vi "Lab Panel V5.28.vi"() -> ()   [LabVIEW 2013] (continued)
                            n2525 = Build Array("AMPS ON", "AMPS OFF", "VOLTS", "PF", "TEMP Live", "TEMP Neut", "CYCLE") -> (w4589:string[])
                            n2526 = Bundle By Name("Y"=w4612, "t0"=w4605) -> (w4604:waveform(dbl))  [unwired: 1 in]
                            n2527 = Bundle By Name("Y"=w4611, "t0"=w4605) -> (w4603:waveform(dbl))  [unwired: 1 in]
                            n2528 = Bundle By Name("Y"=w4610, "t0"=w4605) -> (w4602:waveform(dbl))  [unwired: 1 in]
                            n2529 = Bundle By Name("Y"=w4609, "t0"=w4605) -> (w4601:waveform(dbl))  [unwired: 1 in]
                            n2530 = Bundle By Name("Y"=w4608, "t0"=w4605) -> (w4600:waveform(dbl))  [unwired: 1 in]
                            n2531 = Bundle By Name("Y"=w4607, "t0"=w4605) -> (w4599:waveform(dbl))  [unwired: 1 in]
                            n2532 = Bundle By Name("Y"=w4606, "t0"=w4605) -> (w4598:waveform(dbl))  [unwired: 1 in]
                            n2533 = Build Array(w4604, w4603, w4602, w4601, w4600, w4599, w4598) -> (w4597:waveform(dbl)[])
                            n2534 = TDMS Write(0:w4618, 5:"TEST VALUES", 7:w4589, 9:w4597) -> (4:w4588:refnum<k34>, 6:w4587:string, 15:w4586:errorcluster)  [unwired: 2 in, 1 out]
                            n2535 = TDMS Write(0:w4588, 5:w4587, 7:"TIME", 9:w4584, 11:w4586) -> (15:w4583:errorcluster)  [unwired: 1 in, 3 out]
                            n2536 = local write "data file error"(w4583) -> ()
                          }
                        }
                      }
                    }
                  }
                }
              }
              frame #8 {
                n2537 = case shown="True" w4622 {
                  tunnel: w4626 -> [_ w4631]
                  tunnel: w4625 -> [_ w4630]
                  tunnel: w4624 -> [_ w4628]
                  tunnel: w4623 -> [_ w4627]
                  frame False {
                  }
                  frame True {
                    n2538 = local read "DISP LAB05-1"() -> (w4632:T4)
                    n2539 = local read "SIG LAB05-1"() -> (w4633:T2)
                    n2540 = local read "ON L05-1"() -> (w4629:cluster{"amps":dbl, "volts":dbl, "pf":dbl})
                    n2541 = Unbundle(w4633) -> ("AMPS"=w4639:dbl, "VOLTS"=w4637:dbl, "PF"=w4636:dbl, "Tmp Live"=w4635:dbl, "Tmp Neut"=w4638:dbl)
                    n2542 = Unbundle(w4632) -> ("CYCLE"=w4634:dbl)  [unwired: 2 out]
                    n2543 = stacked-sequence {
                      tunnel: w4639 -> [w4643 w4662]
                      tunnel: w4638 -> [_ w4661]
                      tunnel: w4637 -> [w4642 w4660]
                      tunnel: w4636 -> [w4641 w4659]
                      tunnel: w4635 -> [_ w4658]
                      tunnel: w4634 -> [_ w4657]
                      tunnel: w4631 -> [_ w4656]
                      tunnel: w4630 -> [w4644 _]
                      tunnel: w4629 -> [w4640 w4654]
                      tunnel: w4628 -> [_ w4655]
                      tunnel: w4627 -> [_ w4650]
                      frame #0 {
                        n2544 = case shown="True" w4644 {
                          tunnel: w4643 -> [_ w4649]
                          tunnel: w4642 -> [_ w4648]
                          tunnel: w4641 -> [_ w4647]
                          tunnel: w4640 -> [_ w4645]
                          frame False {
                          }
                          frame True {
                            n2545 = Bundle(cluster=w4645, "amps"=w4649, "volts"=w4648, "pf"=w4647) -> (w4646:cluster{"amps":dbl, "volts":dbl, "pf":dbl})
                            n2546 = local write "ON L05-1"(w4646) -> ()
                          }
                        }
                      }
                      frame #1 {
                        n2547 = Unbundle(w4654) -> ("amps"=w4653:dbl, "volts"=w4652:dbl, "pf"=w4651:dbl)
                        n2548 = case shown="True" w4655 {
                          tunnel: w4662 -> [_ w4694]
                          tunnel: w4661 -> [_ w4701]
                          tunnel: w4660 -> [_ _]
                          tunnel: w4659 -> [_ _]
                          tunnel: w4658 -> [_ w4700]
                          tunnel: w4657 -> [_ w4699]
                          tunnel: w4656 -> [_ w4664]
                          tunnel: w4653 -> [_ w4696]
                          tunnel: w4652 -> [_ w4695]
                          tunnel: w4651 -> [_ w4693]
                          tunnel: w4650 -> [_ w4685]
                          frame False {
                          }
                          frame True {
                            n2549 = local read "TDMS LAB05-1"() -> (w4698:refnum<k34>)
                            n2550 = Build Array(w4695) -> (w4690:dbl[])
                            n2551 = Build Array(w4693) -> (w4689:dbl[])
                            n2552 = Build Array(w4700) -> (w4688:dbl[])
                            n2553 = Build Array(w4701) -> (w4687:dbl[])
                            n2554 = Build Array(w4696) -> (w4692:dbl[])
                            n2555 = Build Array(w4694) -> (w4691:dbl[])
                            n2556 = Build Array(w4699) -> (w4686:dbl[])
                            n2557 = Build Array("AMPS ON", "AMPS OFF", "VOLTS", "PF", "TEMP Live", "TEMP Neut", "CYCLE") -> (w4669:string[])
                            n2558 = Bundle By Name("Y"=w4692, "t0"=w4685) -> (w4684:waveform(dbl))  [unwired: 1 in]
                            n2559 = Bundle By Name("Y"=w4691, "t0"=w4685) -> (w4683:waveform(dbl))  [unwired: 1 in]
                            n2560 = Bundle By Name("Y"=w4690, "t0"=w4685) -> (w4682:waveform(dbl))  [unwired: 1 in]
                            n2561 = Bundle By Name("Y"=w4689, "t0"=w4685) -> (w4681:waveform(dbl))  [unwired: 1 in]
                            n2562 = Bundle By Name("Y"=w4688, "t0"=w4685) -> (w4680:waveform(dbl))  [unwired: 1 in]
                            n2563 = Bundle By Name("Y"=w4687, "t0"=w4685) -> (w4679:waveform(dbl))  [unwired: 1 in]
                            n2564 = Bundle By Name("Y"=w4686, "t0"=w4685) -> (w4678:waveform(dbl))  [unwired: 1 in]
                            n2565 = Build Array(w4684, w4683, w4682, w4681, w4680, w4679, w4678) -> (w4677:waveform(dbl)[])
                            n2566 = TDMS Write(0:w4698, 5:"TEST VALUES", 7:w4669, 9:w4677) -> (4:w4668:refnum<k34>, 6:w4667:string, 15:w4666:errorcluster)  [unwired: 2 in, 1 out]
                            n2567 = TDMS Write(0:w4668, 5:w4667, 7:"TIME", 9:w4664, 11:w4666) -> (15:w4663:errorcluster)  [unwired: 1 in, 3 out]
                            n2568 = local write "data file error"(w4663) -> ()
                          }
                        }
                      }
                    }
                  }
                }
              }
              frame #9 {
                n2569 = case shown="True" w4702 {
                  tunnel: w4706 -> [_ w4711]
                  tunnel: w4705 -> [_ w4710]
                  tunnel: w4704 -> [_ w4708]
                  tunnel: w4703 -> [_ w4707]
                  frame False {
                  }
                  frame True {
                    n2570 = local read "DISP LAB05-2"() -> (w4712:T4)
                    n2571 = local read "SIG LAB05-2"() -> (w4713:T2)
                    n2572 = local read "ON L05-2"() -> (w4709:cluster{"amps":dbl, "volts":dbl, "pf":dbl})
                    n2573 = Unbundle(w4713) -> ("AMPS"=w4719:dbl, "VOLTS"=w4717:dbl, "PF"=w4716:dbl, "Tmp Live"=w4715:dbl, "Tmp Neut"=w4718:dbl)
                    n2574 = Unbundle(w4712) -> ("CYCLE"=w4714:dbl)  [unwired: 2 out]
                    n2575 = stacked-sequence {
                      tunnel: w4719 -> [w4723 w4742]
                      tunnel: w4718 -> [_ w4741]
                      tunnel: w4717 -> [w4722 w4740]
                      tunnel: w4716 -> [w4721 w4739]
                      tunnel: w4715 -> [_ w4738]
                      tunnel: w4714 -> [_ w4737]
                      tunnel: w4711 -> [_ w4736]
                      tunnel: w4710 -> [w4724 _]
                      tunnel: w4709 -> [w4720 w4734]
                      tunnel: w4708 -> [_ w4735]
                      tunnel: w4707 -> [_ w4730]
                      frame #0 {
                        n2576 = case shown="True" w4724 {
                          tunnel: w4723 -> [_ w4729]
                          tunnel: w4722 -> [_ w4728]
                          tunnel: w4721 -> [_ w4727]
                          tunnel: w4720 -> [_ w4725]
                          frame False {
                          }
                          frame True {
                            n2577 = Bundle(cluster=w4725, "amps"=w4729, "volts"=w4728, "pf"=w4727) -> (w4726:cluster{"amps":dbl, "volts":dbl, "pf":dbl})
                            n2578 = local write "ON L05-2"(w4726) -> ()
                          }
                        }
                      }
                      frame #1 {
                        n2579 = Unbundle(w4734) -> ("amps"=w4733:dbl, "volts"=w4732:dbl, "pf"=w4731:dbl)
                        n2580 = case shown="True" w4735 {
                          tunnel: w4742 -> [_ w4774]
                          tunnel: w4741 -> [_ w4781]
                          tunnel: w4740 -> [_ _]
                          tunnel: w4739 -> [_ _]
                          tunnel: w4738 -> [_ w4780]
                          tunnel: w4737 -> [_ w4779]
                          tunnel: w4736 -> [_ w4744]
                          tunnel: w4733 -> [_ w4776]
                          tunnel: w4732 -> [_ w4775]
                          tunnel: w4731 -> [_ w4773]
                          tunnel: w4730 -> [_ w4765]
                          frame False {
                          }
                          frame True {
                            n2581 = local read "TDMS LAB05-2"() -> (w4778:refnum<k34>)
                            n2582 = Build Array(w4775) -> (w4770:dbl[])
                            n2583 = Build Array(w4773) -> (w4769:dbl[])
                            n2584 = Build Array(w4780) -> (w4768:dbl[])
                            n2585 = Build Array(w4781) -> (w4767:dbl[])
                            n2586 = Build Array(w4776) -> (w4772:dbl[])
                            n2587 = Build Array(w4774) -> (w4771:dbl[])
                            n2588 = Build Array(w4779) -> (w4766:dbl[])
                            n2589 = Build Array("AMPS ON", "AMPS OFF", "VOLTS", "PF", "TEMP Live", "TEMP Neut", "CYCLE") -> (w4749:string[])
                            n2590 = Bundle By Name("Y"=w4772, "t0"=w4765) -> (w4764:waveform(dbl))  [unwired: 1 in]
                            n2591 = Bundle By Name("Y"=w4771, "t0"=w4765) -> (w4763:waveform(dbl))  [unwired: 1 in]
                            n2592 = Bundle By Name("Y"=w4770, "t0"=w4765) -> (w4762:waveform(dbl))  [unwired: 1 in]
                            n2593 = Bundle By Name("Y"=w4769, "t0"=w4765) -> (w4761:waveform(dbl))  [unwired: 1 in]
                            n2594 = Bundle By Name("Y"=w4768, "t0"=w4765) -> (w4760:waveform(dbl))  [unwired: 1 in]
                            n2595 = Bundle By Name("Y"=w4767, "t0"=w4765) -> (w4759:waveform(dbl))  [unwired: 1 in]
                            n2596 = Bundle By Name("Y"=w4766, "t0"=w4765) -> (w4758:waveform(dbl))  [unwired: 1 in]
                            n2597 = Build Array(w4764, w4763, w4762, w4761, w4760, w4759, w4758) -> (w4757:waveform(dbl)[])
                            n2598 = TDMS Write(0:w4778, 5:"TEST VALUES", 7:w4749, 9:w4757) -> (4:w4748:refnum<k34>, 6:w4747:string, 15:w4746:errorcluster)  [unwired: 2 in, 1 out]
                            n2599 = TDMS Write(0:w4748, 5:w4747, 7:"TIME", 9:w4744, 11:w4746) -> (15:w4743:errorcluster)  [unwired: 1 in, 3 out]
                            n2600 = local write "data file error"(w4743) -> ()
                          }
                        }
                      }
                    }
                  }
                }
              }
            }
          }
          frame #15 {
            # "display test values on chart"
            n2601 = local read "jig cycle"() -> (w4786:dbl)
            n2602 = local read "on loops"() -> (w4788:dbl)
            n2603 = Add(x=w4788, y=4) -> (x+y=w4785:dbl)
            n2604 = Equal?(x=w4786, y=3) -> (x = y?=w4784:bool)
            n2605 = Equal?(x=w4786, y=w4785) -> (x = y?=w4783:bool)
            n2606 = Or(x=w4784, y=w4783) -> (x .or. y?=w4782:bool)
            "graph flag" <- w4782
            n2607 = global write "Global display 3.vi" "graph flag"(w4782) -> ()
            n2608 = case shown="True" w4782 {
              frame False {
              }
              frame True {
                n2609 = local read "SIG LAB05-1"() -> (w4831:T2)
                n2610 = local read "SIG LAB04-2"() -> (w4832:T2)
                n2611 = local read "SIG LAB05-2"() -> (w4830:T2)
                n2612 = local read "SIG LAB04-1"() -> (w4833:T2)
                n2613 = local read "SIG LAB03-1"() -> (w4835:T2)
                n2614 = local read "SIG LAB03-2"() -> (w4834:T2)
                n2615 = local read "SIG LAB01-1"() -> (w4839:T2)
                n2616 = local read "SIG LAB02-2"() -> (w4836:T2)
                n2617 = local read "SIG LAB02-1"() -> (w4837:T2)
                n2618 = local read "SIG LAB01-2"() -> (w4838:T2)
                n2619 = Unbundle(w4832) -> ("AMPS"=w4822:dbl, "VOLTS"=w4812:dbl, "Tmp Live"=w4802:dbl, "Tmp Neut"=w4792:dbl)  [unwired: 1 out]
                n2620 = Unbundle(w4831) -> ("AMPS"=w4821:dbl, "VOLTS"=w4811:dbl, "Tmp Live"=w4801:dbl, "Tmp Neut"=w4791:dbl)  [unwired: 1 out]
                n2621 = Unbundle(w4830) -> ("AMPS"=w4820:dbl, "VOLTS"=w4810:dbl, "Tmp Live"=w4800:dbl, "Tmp Neut"=w4790:dbl)  [unwired: 1 out]
                n2622 = Unbundle(w4833) -> ("AMPS"=w4823:dbl, "VOLTS"=w4813:dbl, "Tmp Live"=w4803:dbl, "Tmp Neut"=w4793:dbl)  [unwired: 1 out]
                n2623 = Unbundle(w4834) -> ("AMPS"=w4824:dbl, "VOLTS"=w4814:dbl, "Tmp Live"=w4804:dbl, "Tmp Neut"=w4794:dbl)  [unwired: 1 out]
                n2624 = Unbundle(w4835) -> ("AMPS"=w4825:dbl, "VOLTS"=w4815:dbl, "Tmp Live"=w4805:dbl, "Tmp Neut"=w4795:dbl)  [unwired: 1 out]
                n2625 = Unbundle(w4836) -> ("AMPS"=w4826:dbl, "VOLTS"=w4816:dbl, "Tmp Live"=w4806:dbl, "Tmp Neut"=w4796:dbl)  [unwired: 1 out]
                n2626 = Unbundle(w4837) -> ("AMPS"=w4827:dbl, "VOLTS"=w4817:dbl, "Tmp Live"=w4807:dbl, "Tmp Neut"=w4797:dbl)  [unwired: 1 out]
                n2627 = Unbundle(w4839) -> ("AMPS"=w4829:dbl, "VOLTS"=w4819:dbl, "Tmp Live"=w4809:dbl, "Tmp Neut"=w4799:dbl)  [unwired: 1 out]
                n2628 = Unbundle(w4838) -> ("AMPS"=w4828:dbl, "VOLTS"=w4818:dbl, "Tmp Live"=w4808:dbl, "Tmp Neut"=w4798:dbl)  [unwired: 1 out]
                n2629 = stacked-sequence {
                  tunnel: w4829 -> [w4871 _ _]
                  tunnel: w4828 -> [w4870 _ _]
                  tunnel: w4827 -> [w4861 _ _]
                  tunnel: w4826 -> [w4860 _ _]
                  tunnel: w4825 -> [w4850 _ _]
                  tunnel: w4824 -> [w4849 _ _]
                  tunnel: w4823 -> [_ w4894 _]
                  tunnel: w4822 -> [_ w4893 _]
                  tunnel: w4821 -> [_ w4883 _]
                  tunnel: w4820 -> [_ w4882 _]
                  tunnel: w4819 -> [w4868 _ _]
                  tunnel: w4818 -> [w4867 _ _]
                  tunnel: w4817 -> [w4858 _ _]
                  tunnel: w4816 -> [w4857 _ _]
                  tunnel: w4815 -> [w4848 _ _]
                  tunnel: w4814 -> [w4847 _ _]
                  tunnel: w4813 -> [_ w4892 _]
                  tunnel: w4812 -> [_ w4891 _]
                  tunnel: w4811 -> [_ w4881 _]
                  tunnel: w4810 -> [_ w4880 _]
                  tunnel: w4809 -> [w4865 _ _]
                  tunnel: w4808 -> [w4863 _ _]
                  tunnel: w4807 -> [w4854 _ _]
                  tunnel: w4806 -> [w4852 _ _]
                  tunnel: w4805 -> [w4846 _ _]
                  tunnel: w4804 -> [w4844 _ _]
                  tunnel: w4803 -> [_ w4890 _]
                  tunnel: w4802 -> [_ w4888 _]
                  tunnel: w4801 -> [_ w4879 _]
                  tunnel: w4800 -> [_ w4877 _]
                  tunnel: w4799 -> [w4864 _ _]
                  tunnel: w4798 -> [w4862 _ _]
                  tunnel: w4797 -> [w4853 _ _]
                  tunnel: w4796 -> [w4851 _ _]
                  tunnel: w4795 -> [w4845 _ _]
                  tunnel: w4794 -> [w4843 _ _]
                  tunnel: w4793 -> [_ w4889 _]
                  tunnel: w4792 -> [_ w4887 _]
                  tunnel: w4791 -> [_ w4878 _]
                  tunnel: w4790 -> [_ w4876 _]
                  frame #0 {
                    n2630 = Merge Signals(w4871, w4870) -> (→"LAB01 AMPS":dynamicdata)
                    n2631 = Merge Signals(w4868, w4867) -> (→"LAB01 VOLTS":dynamicdata)
                    n2632 = Merge Signals(w4848, w4847) -> (→"LAB03 VOLTS":dynamicdata)
                    n2633 = Merge Signals(w4865, w4864, w4863, w4862) -> (→"LAB01 deg C":dynamicdata)
                    n2634 = Merge Signals(w4861, w4860) -> (→"LAB02 AMPS":dynamicdata)
                    n2635 = Merge Signals(w4854, w4853, w4852, w4851) -> (→"LAB02 deg C":dynamicdata)
                    n2636 = Merge Signals(w4846, w4845, w4844, w4843) -> (→"LAB03 deg C":dynamicdata)
                    n2637 = Merge Signals(w4858, w4857) -> (→"LAB02 VOLTS":dynamicdata)
                    n2638 = Merge Signals(w4850, w4849) -> (→"LAB03 AMPS":dynamicdata)
                  }
                  frame #1 {
                    n2639 = Merge Signals(w4881, w4880) -> (→"LAB05 VOLTS":dynamicdata)
                    n2640 = Merge Signals(w4894, w4893) -> (→"LAB04 AMPS":dynamicdata)
                    n2641 = Merge Signals(w4883, w4882) -> (→"LAB05 AMPS":dynamicdata)
                    n2642 = Merge Signals(w4879, w4878, w4877, w4876) -> (→"LAB05 deg C":dynamicdata)
                    n2643 = Merge Signals(w4890, w4889, w4888, w4887) -> (→"LAB04 deg C":dynamicdata)
                    n2644 = Merge Signals(w4892, w4891) -> (→"LAB04 VOLTS":dynamicdata)
                  }
                  frame #2 {
                    n2645 = local read "LAB05 VOLTS"() -> (w4902:dynamicdata)
                    n2646 = local read "LAB04 VOLTS"() -> (w4903:dynamicdata)
                    n2647 = local read "LAB02 VOLTS"() -> (w4905:dynamicdata)
                    n2648 = local read "LAB03 VOLTS"() -> (w4904:dynamicdata)
                    n2649 = local read "LAB05 AMPS"() -> (w4908:dynamicdata)
                    n2650 = local read "LAB01 VOLTS"() -> (w4906:dynamicdata)
                    n2651 = local read "LAB04 AMPS"() -> (w4909:dynamicdata)
                    n2652 = local read "LAB03 AMPS"() -> (w4910:dynamicdata)
                    n2653 = local read "LAB03 deg C"() -> (w4898:dynamicdata)
                    n2654 = local read "LAB02 AMPS"() -> (w4911:dynamicdata)
                    n2655 = local read "LAB04 deg C"() -> (w4897:dynamicdata)
                    n2656 = local read "LAB05 deg C"() -> (w4896:dynamicdata)
                    n2657 = local read "LAB02 deg C"() -> (w4899:dynamicdata)
                    n2658 = local read "LAB01 deg C"() -> (w4900:dynamicdata)
                    n2659 = local read "LAB01 AMPS"() -> (w4912:dynamicdata)
                    n2660 = Merge Signals(w4900, w4899, w4898, w4897, w4896) -> (w4895:dynamicdata)
                    n2661 = Merge Signals(w4912, w4911, w4910, w4909, w4908) -> (w4907:dynamicdata)
                    n2662 = Merge Signals(w4906, w4905, w4904, w4903, w4902) -> (w4901:dynamicdata)
                    n2663 = global write "Global display 3.vi" "graph volts"(w4901) -> ()
                    n2664 = global write "Global display 3.vi" "graph deg C"(w4895) -> ()
                    n2665 = global write "Global display 3.vi" "graph amps"(w4907) -> ()
                  }
                }
              }
            }
          }
          frame #16 {
            # "check for amps fail"
            # "check for cycle test & temperature rise fail conditions"
            n2666 = local read "on loops"() -> (w4939:dbl)
            n2667 = local read "jig cycle"() -> (w4936:dbl)
            n2668 = local read "jig cycle"() -> (w4941:dbl)
            n2669 = Add(x=w4939, y=5.0) -> (x+y=w4937:dbl)
            n2670 = Equal?(x=w4936, y=w4937) -> (x = y?=w4932:bool)
            n2671 = local read "Fail Loops"() -> (w4913:dbl)
            n2672 = Equal?(x=w4941, y=3.0) -> (x = y?=w4934:bool)
            n2673 = global write "Global 1.vi" "fail count"(w4913) -> ()
            n2674 = stacked-sequence {
              tunnel: w4935 -> [w4944 _ _ _ _ _ _ _ _ _]
              tunnel: w4934 -> [w4945 w4965 w4985 w5005 w5025 w5045 w5065 w5085 w5105 w5125]
              tunnel: w4933 -> [w4942 _ _ _ _ _ _ _ _ _]
              tunnel: w4932 -> [w4943 w4964 w4984 w5004 w5024 w5044 w5064 w5084 w5104 w5124]
              tunnel: w4931 -> [_ w4963 _ _ _ _ _ _ _ _]
              tunnel: w4930 -> [_ w4962 _ _ _ _ _ _ _ _]
              tunnel: w4929 -> [_ _ w4983 _ _ _ _ _ _ _]
              tunnel: w4928 -> [_ _ w4982 _ _ _ _ _ _ _]
              tunnel: w4927 -> [_ _ _ w5003 _ _ _ _ _ _]
              tunnel: w4926 -> [_ _ _ w5002 _ _ _ _ _ _]
              tunnel: w4925 -> [_ _ _ _ w5023 _ _ _ _ _]
              tunnel: w4924 -> [_ _ _ _ w5022 _ _ _ _ _]
              tunnel: w4923 -> [_ _ _ _ _ w5043 _ _ _ _]
              tunnel: w4922 -> [_ _ _ _ _ w5042 _ _ _ _]
              tunnel: w4921 -> [_ _ _ _ _ _ w5063 _ _ _]
              tunnel: w4920 -> [_ _ _ _ _ _ w5062 _ _ _]
              tunnel: w4919 -> [_ _ _ _ _ _ _ w5083 _ _]
              tunnel: w4918 -> [_ _ _ _ _ _ _ w5082 _ _]
              tunnel: w4917 -> [_ _ _ _ _ _ _ _ w5103 _]
              tunnel: w4916 -> [_ _ _ _ _ _ _ _ w5102 _]
              tunnel: w4915 -> [_ _ _ _ _ _ _ _ _ w5123]
              tunnel: w4914 -> [_ _ _ _ _ _ _ _ _ w5122]
              frame #0 {
                # "LAB01-1"
                n2675 = case shown="True" w4942 {
                  tunnel: w4945 -> [_ w4958]
                  tunnel: w4944 -> [_ w4955]
                  tunnel: w4943 -> [_ w4954]
                  frame False {
                  }
                  frame True {
                    n2676 = local read "TEMP START LAB01-1"() -> (w4960:cluster{"TL":dbl, "TN":dbl})
                    n2677 = local read "RESULT LAB01-1"() -> (w4949:bool)
                    n2678 = local read "FAIL LAB01-1"() -> (w4952:cluster{"LO":dbl, "HI":dbl})
                    n2679 = local read "TDMS LAB01-1"() -> (w4959:refnum<k34>)
                    n2680 = local read "SET LAB01-1"() -> (w4956:T5)
                    n2681 = local read "DISP LAB01-1"() -> (w4957:T4)
                    n2682 = local read "SIG LAB01-1"() -> (w4961:T2)
                    n2683 = Bundle("FAIL LAB01-1"=w4952, "SIG LAB01-1"=w4961, "TEMP START LAB01-1"=w4960, "DISP LAB01-1"=w4957, "SET LAB01-1"=w4956, "TDMS LAB01-1"=w4959) -> (w4946:T33)  [unwired: 1 in]
                    n2684 = call "sub vi - cycle&temp fail v7.vi"("Amps Lo?"=w4958, "Input Cluster"=w4946, "SELECT"=w4955, "Amps Hi?"=w4954, "Result In"=w4949) -> ("(FAIL) out"=w4951:cluster{"FAIL LO":dbl, "FAIL HI":dbl}, "(DISP) out"=w4947:T4, "T-RISE"=w4948:cluster{"T-RISE (L)":dbl, "T-RISE (N)":dbl}, "Result Out"=w4950:bool, "file error"=w4953:errorcluster)  [unwired: 10 in]
                    n2685 = local write "TEMP RISE LAB01-1"(w4948) -> ()
                    n2686 = local write "FAIL LAB01-1"(w4951) -> ()
                    n2687 = local write "DISP LAB01-1"(w4947) -> ()
                    n2688 = local write "RESULT LAB01-1"(w4950) -> ()
                    n2689 = local write "data file error"(w4953) -> ()
                  }
                }
              }
              frame #1 {
                # "LAB01-2"
                n2690 = case shown="True" w4963 {
                  tunnel: w4965 -> [_ w4978]
                  tunnel: w4962 -> [_ w4975]
                  tunnel: w4964 -> [_ w4974]
                  frame False {
                  }
                  frame True {
                    n2691 = local read "TEMP START LAB01-2"() -> (w4980:cluster{"TL":dbl, "TN":dbl})
                    n2692 = local read "FAIL LAB01-2"() -> (w4971:cluster{"LO":dbl, "HI":dbl})
                    n2693 = local read "TDMS LAB01-2"() -> (w4979:refnum<k34>)
                    n2694 = local read "SET LAB01-2"() -> (w4976:T5)
                    n2695 = local read "DISP LAB01-2"() -> (w4977:T4)
                    n2696 = local read "RESULT LAB01-2"() -> (w4968:bool)
                    n2697 = local read "SIG LAB01-2"() -> (w4981:T2)
                    n2698 = Bundle("FAIL LAB01-2"=w4971, "SIG LAB01-2"=w4981, "TEMP START LAB01-2"=w4980, "DISP LAB01-2"=w4977, "SET LAB01-2"=w4976, "TDMS LAB01-2"=w4979) -> (w4966:T34)  [unwired: 1 in]
                    n2699 = call "sub vi - cycle&temp fail v7.vi"("Amps Lo?"=w4978, "Input Cluster"=w4966, "SELECT"=w4975, "Amps Hi?"=w4974, "Result In"=w4968) -> ("(FAIL) out"=w4970:cluster{"FAIL LO":dbl, "FAIL HI":dbl}, "(DISP) out"=w4973:T4, "T-RISE"=w4967:cluster{"T-RISE (L)":dbl, "T-RISE (N)":dbl}, "Result Out"=w4969:bool, "file error"=w4972:errorcluster)  [unwired: 10 in]
                    n2700 = local write "TEMP RISE LAB01-2"(w4967) -> ()
                    n2701 = local write "FAIL LAB01-2"(w4970) -> ()
                    n2702 = local write "DISP LAB01-2"(w4973) -> ()
                    n2703 = local write "RESULT LAB01-2"(w4969) -> ()
                    n2704 = local write "data file error"(w4972) -> ()
                  }
                }
              }
              frame #2 {
                # "LAB02-1"
                n2705 = case shown="True" w4983 {
                  tunnel: w4985 -> [_ w4998]
                  tunnel: w4982 -> [_ w4995]
                  tunnel: w4984 -> [_ w4994]
                  frame False {
                  }
                  frame True {
                    n2706 = local read "TEMP START LAB02-1"() -> (w5000:cluster{"TL":dbl, "TN":dbl})
                    n2707 = local read "FAIL LAB02-1"() -> (w4991:cluster{"LO":dbl, "HI":dbl})
                    n2708 = local read "TDMS LAB02-1"() -> (w4999:refnum<k34>)
                    n2709 = local read "SET LAB02-1"() -> (w4996:T5)
                    n2710 = local read "DISP LAB02-1"() -> (w4997:T4)
                    n2711 = local read "SIG LAB02-1"() -> (w5001:T2)
                    n2712 = local read "RESULT LAB02-1"() -> (w4988:bool)
                    n2713 = Bundle("FAIL LAB02-1"=w4991, "SIG LAB02-1"=w5001, "TEMP START LAB02-1"=w5000, "DISP LAB02-1"=w4997, "SET LAB02-1"=w4996, "TDMS LAB02-1"=w4999) -> (w4986:T35)  [unwired: 1 in]
                    n2714 = call "sub vi - cycle&temp fail v7.vi"("Amps Lo?"=w4998, "Input Cluster"=w4986, "SELECT"=w4995, "Amps Hi?"=w4994, "Result In"=w4988) -> ("(FAIL) out"=w4990:cluster{"FAIL LO":dbl, "FAIL HI":dbl}, "(DISP) out"=w4993:T4, "T-RISE"=w4987:cluster{"T-RISE (L)":dbl, "T-RISE (N)":dbl}, "Result Out"=w4989:bool, "file error"=w4992:errorcluster)  [unwired: 10 in]
                    n2715 = local write "TEMP RISE LAB02-1"(w4987) -> ()
                    n2716 = local write "FAIL LAB02-1"(w4990) -> ()
                    n2717 = local write "DISP LAB02-1"(w4993) -> ()
                    n2718 = local write "RESULT LAB02-1"(w4989) -> ()
                    n2719 = local write "data file error"(w4992) -> ()
                  }
                }
              }
              frame #3 {
                # "LAB02-2"
                n2720 = case shown="True" w5003 {
                  tunnel: w5005 -> [_ w5018]
                  tunnel: w5002 -> [_ w5015]
                  tunnel: w5004 -> [_ w5014]
                  frame False {
                  }
                  frame True {
                    n2721 = local read "TEMP START LAB02-2"() -> (w5020:cluster{"TL":dbl, "TN":dbl})
                    n2722 = local read "FAIL LAB02-2"() -> (w5011:cluster{"LO":dbl, "HI":dbl})
                    n2723 = local read "TDMS LAB02-2"() -> (w5019:refnum<k34>)
                    n2724 = local read "SET LAB02-2"() -> (w5016:T5)
                    n2725 = local read "DISP LAB02-2"() -> (w5017:T4)
                    n2726 = local read "SIG LAB02-2"() -> (w5021:T2)
                    n2727 = local read "RESULT LAB02-2"() -> (w5008:bool)
                    n2728 = Bundle("FAIL LAB02-2"=w5011, "SIG LAB02-2"=w5021, "TEMP START LAB02-2"=w5020, "DISP LAB02-2"=w5017, "SET LAB02-2"=w5016, "TDMS LAB02-2"=w5019) -> (w5006:T36)  [unwired: 1 in]
                    n2729 = call "sub vi - cycle&temp fail v7.vi"("Amps Lo?"=w5018, "Input Cluster"=w5006, "SELECT"=w5015, "Amps Hi?"=w5014, "Result In"=w5008) -> ("(FAIL) out"=w5010:cluster{"FAIL LO":dbl, "FAIL HI":dbl}, "(DISP) out"=w5013:T4, "T-RISE"=w5007:cluster{"T-RISE (L)":dbl, "T-RISE (N)":dbl}, "Result Out"=w5009:bool, "file error"=w5012:errorcluster)  [unwired: 10 in]
                    n2730 = local write "TEMP RISE LAB02-2"(w5007) -> ()
                    n2731 = local write "FAIL LAB02-2"(w5010) -> ()
                    n2732 = local write "DISP LAB02-2"(w5013) -> ()
                    n2733 = local write "RESULT LAB02-2"(w5009) -> ()
                    n2734 = local write "data file error"(w5012) -> ()
                  }
                }
              }
              frame #4 {
                # "LAB03-1"
                n2735 = case shown="True" w5023 {
                  tunnel: w5025 -> [_ w5038]
                  tunnel: w5022 -> [_ w5035]
                  tunnel: w5024 -> [_ w5034]
                  frame False {
                  }
                  frame True {
                    n2736 = local read "TEMP START LAB03-1"() -> (w5040:cluster{"TL":dbl, "TN":dbl})
                    n2737 = local read "FAIL LAB03-1"() -> (w5031:cluster{"LO":dbl, "HI":dbl})
                    n2738 = local read "TDMS LAB03-1"() -> (w5039:refnum<k34>)
                    n2739 = local read "SET LAB03-1"() -> (w5036:T5)
                    n2740 = local read "DISP LAB03-1"() -> (w5037:T4)
                    n2741 = local read "SIG LAB03-1"() -> (w5041:T2)
                    n2742 = local read "RESULT LAB03-1"() -> (w5028:bool)
                    n2743 = Bundle("FAIL LAB03-1"=w5031, "SIG LAB03-1"=w5041, "TEMP START LAB03-1"=w5040, "DISP LAB03-1"=w5037, "SET LAB03-1"=w5036, "TDMS LAB03-1"=w5039) -> (w5026:T37)  [unwired: 1 in]
                    n2744 = call "sub vi - cycle&temp fail v7.vi"("Amps Lo?"=w5038, "Input Cluster"=w5026, "SELECT"=w5035, "Amps Hi?"=w5034, "Result In"=w5028) -> ("(FAIL) out"=w5030:cluster{"FAIL LO":dbl, "FAIL HI":dbl}, "(DISP) out"=w5033:T4, "T-RISE"=w5027:cluster{"T-RISE (L)":dbl, "T-RISE (N)":dbl}, "Result Out"=w5029:bool, "file error"=w5032:errorcluster)  [unwired: 10 in]
                    n2745 = local write "TEMP RISE LAB03-1"(w5027) -> ()
                    n2746 = local write "FAIL LAB03-1"(w5030) -> ()
                    n2747 = local write "DISP LAB03-1"(w5033) -> ()
                    n2748 = local write "RESULT LAB03-1"(w5029) -> ()
                    n2749 = local write "data file error"(w5032) -> ()
                  }
                }
              }
              frame #5 {
                # "LAB03-2"
                n2750 = case shown="True" w5043 {
                  tunnel: w5045 -> [_ w5058]
                  tunnel: w5042 -> [_ w5055]
                  tunnel: w5044 -> [_ w5054]
                  frame False {
                  }
                  frame True {
                    n2751 = local read "TEMP START LAB03-2"() -> (w5060:cluster{"TL":dbl, "TN":dbl})
                    n2752 = local read "FAIL LAB03-2"() -> (w5051:cluster{"LO":dbl, "HI":dbl})
                    n2753 = local read "TDMS LAB03-2"() -> (w5059:refnum<k34>)
                    n2754 = local read "SET LAB03-2"() -> (w5056:T5)
                    n2755 = local read "DISP LAB03-2"() -> (w5057:T4)
                    n2756 = local read "RESULT LAB03-2"() -> (w5048:bool)
                    n2757 = local read "SIG LAB03-2"() -> (w5061:T2)
                    n2758 = Bundle("FAIL LAB03-2"=w5051, "SIG LAB03-2"=w5061, "TEMP START LAB03-2"=w5060, "DISP LAB03-2"=w5057, "SET LAB03-2"=w5056, "TDMS LAB03-2"=w5059) -> (w5046:T38)  [unwired: 1 in]
                    n2759 = call "sub vi - cycle&temp fail v7.vi"("Amps Lo?"=w5058, "Input Cluster"=w5046, "SELECT"=w5055, "Amps Hi?"=w5054, "Result In"=w5048) -> ("(FAIL) out"=w5050:cluster{"FAIL LO":dbl, "FAIL HI":dbl}, "(DISP) out"=w5053:T4, "T-RISE"=w5047:cluster{"T-RISE (L)":dbl, "T-RISE (N)":dbl}, "Result Out"=w5049:bool, "file error"=w5052:errorcluster)  [unwired: 10 in]
                    n2760 = local write "FAIL LAB03-2"(w5050) -> ()
                    n2761 = local write "TEMP RISE LAB03-2"(w5047) -> ()
                    n2762 = local write "DISP LAB03-2"(w5053) -> ()
                    n2763 = local write "RESULT LAB03-2"(w5049) -> ()
                    n2764 = local write "data file error"(w5052) -> ()
                  }
                }
              }
              frame #6 {
                # "LAB04-1"
                n2765 = case shown="True" w5063 {
                  tunnel: w5065 -> [_ w5078]
                  tunnel: w5062 -> [_ w5075]
                  tunnel: w5064 -> [_ w5074]
                  frame False {
                  }
                  frame True {
                    n2766 = local read "TEMP START LAB04-1"() -> (w5080:cluster{"TL":dbl, "TN":dbl})
                    n2767 = local read "FAIL LAB04-1"() -> (w5071:cluster{"LO":dbl, "HI":dbl})
                    n2768 = local read "TDMS LAB04-1"() -> (w5079:refnum<k34>)
                    n2769 = local read "SET LAB04-1"() -> (w5076:T5)
                    n2770 = local read "DISP LAB04-1"() -> (w5077:T4)
                    n2771 = local read "SIG LAB04-1"() -> (w5081:T2)
                    n2772 = local read "RESULT LAB04-1"() -> (w5068:bool)
                    n2773 = Bundle("FAIL LAB04-1"=w5071, "SIG LAB04-1"=w5081, "TEMP START LAB04-1"=w5080, "DISP LAB04-1"=w5077, "SET LAB04-1"=w5076, "TDMS LAB04-1"=w5079) -> (w5066:T39)  [unwired: 1 in]
                    n2774 = call "sub vi - cycle&temp fail v7.vi"("Amps Lo?"=w5078, "Input Cluster"=w5066, "SELECT"=w5075, "Amps Hi?"=w5074, "Result In"=w5068) -> ("(FAIL) out"=w5070:cluster{"FAIL LO":dbl, "FAIL HI":dbl}, "(DISP) out"=w5073:T4, "T-RISE"=w5067:cluster{"T-RISE (L)":dbl, "T-RISE (N)":dbl}, "Result Out"=w5069:bool, "file error"=w5072:errorcluster)  [unwired: 10 in]
                    n2775 = local write "TEMP RISE LAB04-1"(w5067) -> ()
                    n2776 = local write "FAIL LAB04-1"(w5070) -> ()
                    n2777 = local write "DISP LAB04-1"(w5073) -> ()
                    n2778 = local write "RESULT LAB04-1"(w5069) -> ()
                    n2779 = local write "data file error"(w5072) -> ()
                  }
                }
              }
              frame #7 {
                # "LAB04-2"
                n2780 = case shown="True" w5083 {
                  tunnel: w5085 -> [_ w5098]
                  tunnel: w5082 -> [_ w5095]
                  tunnel: w5084 -> [_ w5094]
                  frame False {
                  }
                  frame True {
                    n2781 = local read "TEMP START LAB04-2"() -> (w5100:cluster{"TL":dbl, "TN":dbl})
                    n2782 = local read "FAIL LAB04-2"() -> (w5091:cluster{"LO":dbl, "HI":dbl})
                    n2783 = local read "TDMS LAB04-2"() -> (w5099:refnum<k34>)
                    n2784 = local read "SET LAB04-2"() -> (w5096:T5)
                    n2785 = local read "DISP LAB04-2"() -> (w5097:T4)
                    n2786 = local read "SIG LAB04-2"() -> (w5101:T2)
                    n2787 = local read "RESULT LAB04-2"() -> (w5088:bool)
                    n2788 = Bundle("FAIL LAB04-2"=w5091, "SIG LAB04-2"=w5101, "TEMP START LAB04-2"=w5100, "DISP LAB04-2"=w5097, "SET LAB04-2"=w5096, "TDMS LAB04-2"=w5099) -> (w5086:T40)  [unwired: 1 in]
                    n2789 = call "sub vi - cycle&temp fail v7.vi"("Amps Lo?"=w5098, "Input Cluster"=w5086, "SELECT"=w5095, "Amps Hi?"=w5094, "Result In"=w5088) -> ("(FAIL) out"=w5090:cluster{"FAIL LO":dbl, "FAIL HI":dbl}, "(DISP) out"=w5093:T4, "T-RISE"=w5087:cluster{"T-RISE (L)":dbl, "T-RISE (N)":dbl}, "Result Out"=w5089:bool, "file error"=w5092:errorcluster)  [unwired: 10 in]
                    n2790 = local write "TEMP RISE LAB04-2"(w5087) -> ()
                    n2791 = local write "FAIL LAB04-2"(w5090) -> ()
                    n2792 = local write "DISP LAB04-2"(w5093) -> ()
                    n2793 = local write "RESULT LAB04-2"(w5089) -> ()
                    n2794 = local write "data file error"(w5092) -> ()
                  }
                }
              }
              frame #8 {
                # "LAB05-1"
                n2795 = case shown="True" w5103 {
                  tunnel: w5105 -> [_ w5118]
                  tunnel: w5102 -> [_ w5115]
                  tunnel: w5104 -> [_ w5114]
                  frame False {
                  }
                  frame True {
                    n2796 = local read "TEMP START LAB05-1"() -> (w5120:cluster{"TL":dbl, "TN":dbl})
                    n2797 = local read "FAIL LAB05-1"() -> (w5111:cluster{"LO":dbl, "HI":dbl})
                    n2798 = local read "TDMS LAB05-1"() -> (w5119:refnum<k34>)
                    n2799 = local read "SET LAB05-1"() -> (w5116:T5)
                    n2800 = local read "DISP LAB05-1"() -> (w5117:T4)
                    n2801 = local read "SIG LAB05-1"() -> (w5121:T2)
                    n2802 = local read "RESULT LAB05-1"() -> (w5108:bool)
                    n2803 = Bundle("FAIL LAB05-1"=w5111, "SIG LAB05-1"=w5121, "TEMP START LAB05-1"=w5120, "DISP LAB05-1"=w5117, "SET LAB05-1"=w5116, "TDMS LAB05-1"=w5119) -> (w5106:T41)  [unwired: 1 in]
                    n2804 = call "sub vi - cycle&temp fail v7.vi"("Amps Lo?"=w5118, "Input Cluster"=w5106, "SELECT"=w5115, "Amps Hi?"=w5114, "Result In"=w5108) -> ("(FAIL) out"=w5110:cluster{"FAIL LO":dbl, "FAIL HI":dbl}, "(DISP) out"=w5113:T4, "T-RISE"=w5107:cluster{"T-RISE (L)":dbl, "T-RISE (N)":dbl}, "Result Out"=w5109:bool, "file error"=w5112:errorcluster)  [unwired: 10 in]
                    n2805 = local write "TEMP RISE LAB05-1"(w5107) -> ()
                    n2806 = local write "FAIL LAB05-1"(w5110) -> ()
                    n2807 = local write "DISP LAB05-1"(w5113) -> ()
                    n2808 = local write "RESULT LAB05-1"(w5109) -> ()
                    n2809 = local write "data file error"(w5112) -> ()
                  }
                }
              }
              frame #9 {
                # "LAB05-2"
                n2810 = case shown="True" w5123 {
                  tunnel: w5125 -> [_ w5138]
                  tunnel: w5122 -> [_ w5135]
                  tunnel: w5124 -> [_ w5134]
                  frame False {
                  }
                  frame True {
                    n2811 = local read "TEMP START LAB05-2"() -> (w5140:cluster{"TL":dbl, "TN":dbl})
                    n2812 = local read "FAIL LAB05-2"() -> (w5131:cluster{"LO":dbl, "HI":dbl})
                    n2813 = local read "TDMS LAB05-2"() -> (w5139:refnum<k34>)
                    n2814 = local read "SET LAB05-2"() -> (w5136:T5)
                    n2815 = local read "DISP LAB05-2"() -> (w5137:T4)
                    n2816 = local read "SIG LAB05-2"() -> (w5141:T2)
                    n2817 = local read "RESULT LAB05-2"() -> (w5128:bool)
                    n2818 = Bundle("FAIL LAB05-2"=w5131, "SIG LAB05-2"=w5141, "TEMP START LAB05-2"=w5140, "DISP LAB05-2"=w5137, "SET LAB05-2"=w5136, "TDMS LAB05-2"=w5139) -> (w5126:T42)  [unwired: 1 in]
                    n2819 = call "sub vi - cycle&temp fail v7.vi"("Amps Lo?"=w5138, "Input Cluster"=w5126, "SELECT"=w5135, "Amps Hi?"=w5134, "Result In"=w5128) -> ("(FAIL) out"=w5130:cluster{"FAIL LO":dbl, "FAIL HI":dbl}, "(DISP) out"=w5133:T4, "T-RISE"=w5127:cluster{"T-RISE (L)":dbl, "T-RISE (N)":dbl}, "Result Out"=w5129:bool, "file error"=w5132:errorcluster)  [unwired: 10 in]
                    n2820 = local write "TEMP RISE LAB05-2"(w5127) -> ()
                    n2821 = local write "FAIL LAB05-2"(w5130) -> ()
                    n2822 = local write "DISP LAB05-2"(w5133) -> ()
                    n2823 = local write "RESULT LAB05-2"(w5129) -> ()
                    n2824 = local write "data file error"(w5132) -> ()
                  }
                }
              }
            }
          }
          frame #17 {
            # "run calibration routine"
            n2825 = local read "SET (cal)"() -> (w5142:bool)
            n2826 = case shown="True" w5142 {
              frame False {
              }
              frame True {
                n2827 = stacked-sequence {
                  seq-local: [w5143 _ _] -> [_ w5145 _]
                  frame #0 {
                    n2828 = call "CALIBRATION PASSWORD"() -> ("PASSWORD"=w5143:string)  [unwired: 17 in, 2 out]
                  }
                  frame #1 {
                    n2829 = Equal?(x=w5145, y="7777") -> (x = y?=w5144:bool)
                    n2830 = case shown="True" w5144 {
                      frame False {
                      }
                      frame True {
                        n2831 = stacked-sequence {
                          frame #0 {
                            n2832 = local read "SAMPLES"() -> (w5147:dbl)
                            n2833 = local read "AI Task2"() -> (w5148:dbl)
                            n2834 = local read "AI Task1"() -> (w5149:dbl)
                            n2835 = local read "AI Task0"() -> (w5150:dbl)
                            n2836 = local read "Temp Test Cal"() -> (w5151:dbl)
                            n2837 = call "sub vi - calibration v2.vi"("Samples"=w5147, "Task2"=w5148, "Task1"=w5149, "Task0"=w5150, "Temp Test Cal"=w5151) -> ()  [unwired: 7 in]
                          }
                          frame #1 {
                            n2838 = call "sub vi - get calibration values v1.vi"() -> ("TEMP REF CAL"=w5152:dbl, "LAB01 (CAL)"=w5157:T14, "LAB02 (CAL)"=w5156:T15, "LAB03 (CAL)"=w5155:T14, "LAB04 (CAL)"=w5154:T14, "calibration file error out"=w5158:errorcluster, "LAB05 (CAL)"=w5153:T14)  [unwired: 9 in]
                            n2839 = local write "TEMP REF cal"(w5152) -> ()
                            n2840 = local write "cal file error out"(w5158) -> ()
                            n2841 = local write "CAL LAB04"(w5154) -> ()
                            n2842 = local write "CAL LAB05"(w5153) -> ()
                            n2843 = local write "CAL LAB01"(w5157) -> ()
                            n2844 = local write "CAL LAB02"(w5156) -> ()
                            n2845 = local write "CAL LAB03"(w5155) -> ()
                          }
                        }
                      }
                    }
                  }
                  frame #2 {
                    n2846 = local write "SET (cal)"(FALSE) -> ()
                  }
                }
              }
            }
          }
          frame #18 {
            # "save certain settings to file"
            n2847 = String To Path(string="c:\\crabtree\\Set Up\\") -> (path=w5161:path)
            n2848 = Build Path(base path=w5161, name or relative path="settings.bin") -> (appended path=w5163:path)
            n2849 = Build Path(base path=w5161, name or relative path="mail.bin") -> (appended path=w5160:path)
            n2850 = Create Folder(path (use dialog)=w5161) -> (error out=w5166:errorcluster)  [unwired: 2 in, 2 out]
            n2851 = call <vilib>:"Clear Errors.vi"("error in (no error)"=w5166) -> ()  [unwired: 6 in, 1 out]
            n2852 = stacked-sequence {
              seq-local: [w5178 _] -> [_ w5191]
              tunnel: w5163 -> [_ w5192]
              tunnel: w5160 -> [_ w5190]
              frame #0 {
                n2853 = local read "C drive data root dir"() -> (w5177:path)
                n2854 = local read "Select COM port"() -> (w5174:refnum<visa-resource-name>)
                n2855 = local read "Network Directory"() -> (w5183:path)
                n2856 = local read "SET LAB05-2"() -> (w5182:T5)
                n2857 = local read "SET LAB05-1"() -> (w5181:T5)
                n2858 = local read "SET LAB04-2"() -> (w5180:T5)
                n2859 = local read "SET LAB03-2"() -> (w5184:T5)
                n2860 = local read "SET LAB04-1"() -> (w5179:T5)
                n2861 = local read "SET LAB03-1"() -> (w5185:T5)
                n2862 = local read "SET LAB02-2"() -> (w5186:T5)
                n2863 = local read "SET LAB02-1"() -> (w5187:T5)
                n2864 = local read "Temp Delay Lps"() -> (w5173:dbl)
                n2865 = local read "Amps Fail level"() -> (w5169:dbl)
                n2866 = local read "SET LAB01-2"() -> (w5188:T5)
                n2867 = local read "Temp Test Cal"() -> (w5170:dbl)
                n2868 = local read "SET LAB01-1"() -> (w5189:T5)
                n2869 = local read "Mail Test File To:"() -> (w5168:string)
                n2870 = local read "Temp Value"() -> (w5172:dbl)
                n2871 = local read "Fail Loops"() -> (w5171:dbl)
                n2872 = local read "Mail Test Fail"() -> (w5167:bool)
                n2873 = local read "RATE (Hz)"() -> (w5176:dbl)
                n2874 = local read "SAMPLES"() -> (w5175:dbl)
                n2875 = Bundle("SET LAB01-1"=w5189, "SET LAB01-2"=w5188, "SET LAB02-1"=w5187, "SET LAB02-2"=w5186, "SET LAB03-1"=w5185, "SET LAB03-2"=w5184, "SET LAB04-1"=w5179, "SET LAB04-2"=w5180, "SET LAB05-1"=w5181, "SET LAB05-2"=w5182, "Network Directory"=w5183, "C drive data root dir"=w5177, "RATE (Hz)"=w5176, "SAMPLES"=w5175, "Select COM port"=w5174, "Temp Delay Lps"=w5173, "Temp Value"=w5172, "Fail Loops"=w5171, "Temp Test Cal"=w5170, "Amps Fail level"=w5169, "Mail Test File To:"=w5168, "Mail Test Fail"=w5167) -> (w5178:T22)  [unwired: 1 in]
              }
              frame #1 {
                n2876 = event shown="[1] \"SET LAB01-1\", \"SET LAB01-2\", \"SET LAB02-1\", \"SET LAB02-2\", \"SET LAB03-1\", \"SET LAB03-2\", \"SET LAB04-1\", \"SET LAB04-2\", \"SET LAB05-1\", \"SET LAB05-2\", \"Network Directory\", \"C drive data root dir\", \"RATE (Hz)\", \"SAMPLES\", \"Select COM port\", \"Temp Delay Lps\", \"Temp Value\", \"Fail Loops\", \"Temp Test Cal\", \"Amps Fail level\", \"Mail Test File To:\", \"Mail Test Fail\": Value Change" {
                  selector: _ -> [_ _ _]
                  dyn-events: _ -> [_ _ _]
                  timeout: 10.0 -> [_ _ _]
                  tunnel: w5192 -> [_ w5194 _]
                  tunnel: w5191 -> [_ w5195 _]
                  tunnel: w5190 -> [_ _ w5206]
                  event Timeout {
                    n2877 = event-data() -> ()  [unwired: 1 in, 3 out]
                  }
                  event "SET LAB01-1", "SET LAB01-2", "SET LAB02-1", "SET LAB02-2", "SET LAB03-1", "SET LAB03-2", "SET LAB04-1", "SET LAB04-2", "SET LAB05-1", "SET LAB05-2", "Network Directory", "C drive data root dir", "RATE (Hz)", "SAMPLES", "Select COM port", "Temp Delay Lps", "Temp Value", "Fail Loops", "Temp Test Cal", "Amps Fail level", "Mail Test File To:", "Mail Test Fail": Value Change {
                    n2878 = event-data() -> ()  [unwired: 1 in, 6 out]
                    n2879 = Open/Create/Replace File(file path (use dialog)=w5194, operation (0:open)=T17."replace or create") -> (refnum out=w5200:refnum<file>, error out=w5199:errorcluster)  [unwired: 4 in, 1 out]
                    n2880 = Write to Binary File(file (use dialog)=w5200, data=w5195, error in=w5199) -> (refnum out=w5198:refnum<file>, error out=w5197:errorcluster)  [unwired: 3 in, 1 out]
                    n2881 = Close File(refnum=w5198, error in=w5197) -> (error out=w5196:errorcluster)  [unwired: 1 out]
                    n2882 = local write "data file error"(w5196) -> ()
                  }
                  event "MAIL SETTINGS.OUT SERVER ADDRESS", "MAIL SETTINGS.FROM ACCOUNT", "MAIL SETTINGS.USER NAME", "MAIL SETTINGS.PASSWORD", "Auto Mail Send", "TO (string):": Value Change {
                    n2883 = event-data() -> ()  [unwired: 1 in, 6 out]
                    n2884 = local read "MAIL SETTINGS"() -> (w5205:T7)
                    n2885 = local read "Auto Mail Send"() -> (w5203:bool)
                    n2886 = local read "TO (string):"() -> (w5202:string)
                    n2887 = Open/Create/Replace File(file path (use dialog)=w5206, operation (0:open)=T17."replace or create") -> (refnum out=w5211:refnum<file>, error out=w5210:errorcluster)  [unwired: 4 in, 1 out]
                    n2888 = Bundle("MAIL SETTINGS"=w5205, "Auto Mail Send"=w5203, "TO (string):"=w5202) -> (w5204:T43)  [unwired: 1 in]
                    n2889 = Write to Binary File(file (use dialog)=w5211, data=w5204, error in=w5210) -> (refnum out=w5209:refnum<file>, error out=w5208:errorcluster)  [unwired: 3 in, 1 out]
                    n2890 = Close File(refnum=w5209, error in=w5208) -> (error out=w5207:errorcluster)  [unwired: 1 out]
                    n2891 = local write "data file error"(w5207) -> ()
                  }
                }
              }
            }
          }
          frame #19 {
            # "mail control"
            n2892 = local read "MAIL SETTINGS"() -> (w5228:T7)
            n2893 = local read "Auto Mail Send"() -> (w5214:bool)
            n2894 = Unbundle(w5228) -> ("OUT SERVER ADDRESS"=w5227:string, "FROM ACCOUNT"=w5226:string, "TEST MAIL"=w5225:bool)  [unwired: 4 out]
            n2895 = stacked-sequence {
              tunnel: "TO (string):" -> [_ w5267]
              tunnel: w5228 -> [w5233 w5266]
              tunnel: w5227 -> [w5232 w5265]
              tunnel: w5226 -> [w5231 w5264]
              tunnel: w5225 -> [w5230 _]
